vi "Do.vi"(8 "error in (no error)":errorcluster, 10 "Actor in":refnum<class "Actor.lvclass">, 11 "UpdatePV":refnum<class "UpdatePV.lvclass">) -> (0 "error out":errorcluster, 2 "Actor out":refnum<class "Actor.lvclass">)   [LabVIEW 2013, in "CS++DCPwrGui.lvlib" / "UpdatePV.lvclass"]
doc: "(<B>Filename</B>: Actor Framework.lvlib:Message.lvclass:Do.vi)\n\nDefines what a message does when it is received by an actor. Generally, a message instructs an actor to invoke one of its methods.\n\nBy default, this method does nothing. A child class must override it to define behavior. Create a child class by using the Actor Framework Message Maker dialog box."
uses:
  UpdatePV.lvclass
  <vilib>/ActorFramework/Actor/Actor.lvclass
  CS++DCPwrGui/CS++DCPwrGui.lvclass
  CSPP_Core/Actors/CS++PVMonitor Messages/CS++PVUpdate Msg/CS++PVUpdate Msg.lvclass/CS++PVUpdate Msg.ctl
  CSPP_Core/Classes/CS++ProcessVariables/ProcessVariable/PV.lvclass
  CSPP_Core/Actors/CS++PVMonitor Messages/CS++PVUpdate Msg/CS++PVUpdate Msg.lvclass
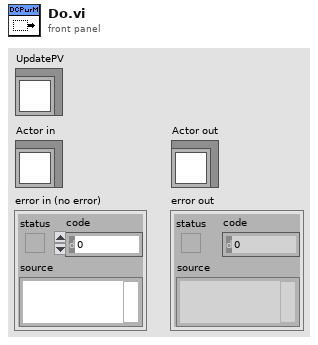
[diagram p1: front panel]
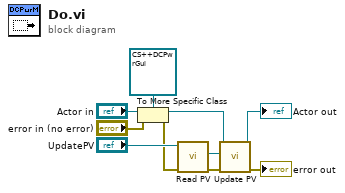
[diagram p0: block diagram]
diagram:
  n1 = To More Specific Class(target class=refnum<class "CS++DCPwrGui.lvclass"> refnum ("CS++DCPwrGui.lvlib:CS++DCPwrGui.lvclass"), reference="Actor in", error in="error in (no error)") -> (specific class reference=w3:refnum<class "CS++DCPwrGui.lvclass">, error out=w4:errorcluster)
  n2 = call "Read PV.vi"("error in (no error)"=w4, "CS++PVUpdate Msg in"="UpdatePV") -> ("error out"=w8:errorcluster, "PV"=w9:refnum<class "PV.lvclass">)  [unwired: 7 in, 1 out]
  n3 = call "Update PV.vi"("error in (no error)"=w8, "PV"=w9, "CS++DCPwrGui in"=w3) -> ("error out"=→"error out":errorcluster, "CS++DCPwrGui out"=→"Actor out":refnum<class "CS++DCPwrGui.lvclass">)  [unwired: 7 in]
